vi "TCP Loop.vi"(8 "error in":errorcluster, 10 "Queues":T1, 11 "Notifiers":T2) -> (0 "error out":errorcluster)   [LabVIEW 2016, in "TCP.lvlib"]
uses:
  TCP.lvlib
  Support/Notifiers/Notifiers.ctl
  Support/Message Queue/All Message Queues.ctl
  Support/Message Queue/Message Cluster.ctl
  TypeDefs/TCP Data.ctl
  Support/Global names.vi
  Support/Message Queue/Enqueue Message (Single).vi
  <vilib>/Utility/error.llb/Error Cluster From Error Code.vi
  <vilib>/ErrorRing/Error Ring.xnode
  support/Message Queue/Message Queue.lvlib
  Model/Model.lvlib
  PLC/PLC.lvlib
  Support/Notifiers/Notifiers.lvlib
panel:
  out "Message":string
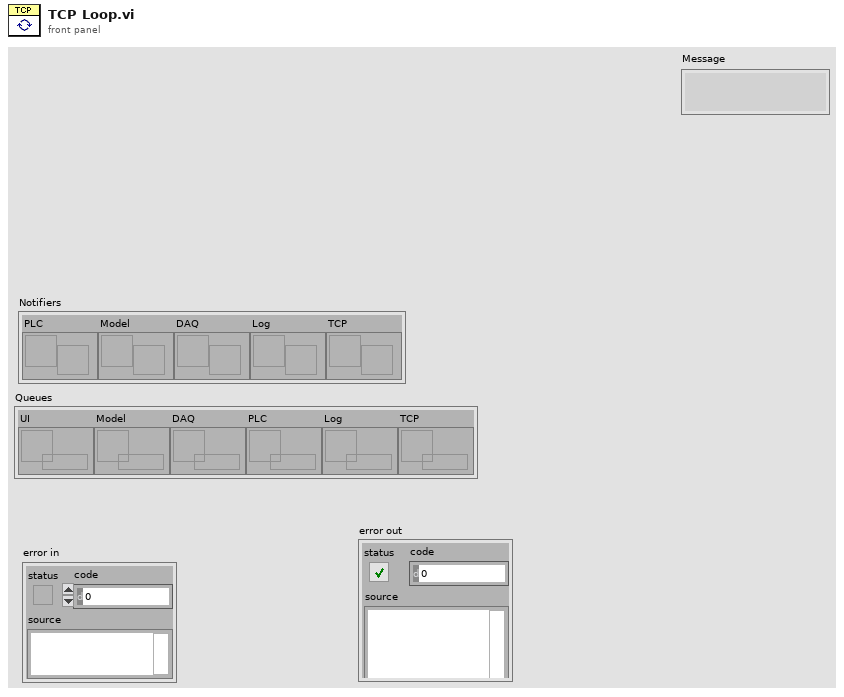
[diagram p1: front panel]
types:
  T1 = typedef "Message Queue.lvlib/All Message Queues.ctl" = cluster{"UI":refnum<queue>, "Model":refnum<queue>, "DAQ":refnum<queue>, "PLC":refnum<queue>, "Log":refnum<queue>, "TCP":refnum<queue>}
  T2 = typedef "Notifiers.lvlib/Notifiers.ctl" = cluster{"PLC":refnum<notifier>, "Model":refnum<notifier>, "DAQ":refnum<notifier>, "Log":refnum<notifier>, "TCP":refnum<notifier>}
  T3 = typedef "TCP.lvlib/TCP Data.ctl" = cluster{"Type":enum16{"Server", "Client"}, "IP":string, "Port":u16, "connection ID":refnum<k5>, "error":errorcluster, "Connected?":bool, "Data":string}
  T4 = enum16{"Standard", "Buffered", "CRLF", "Immediate"}
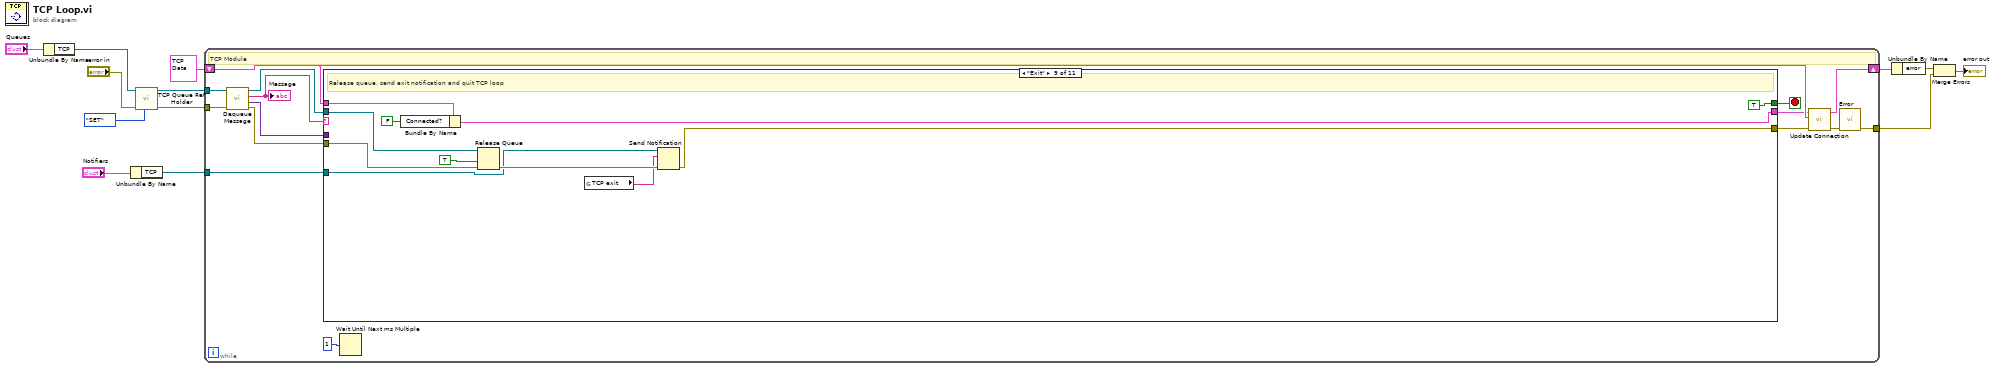
[diagram p0: block diagram]
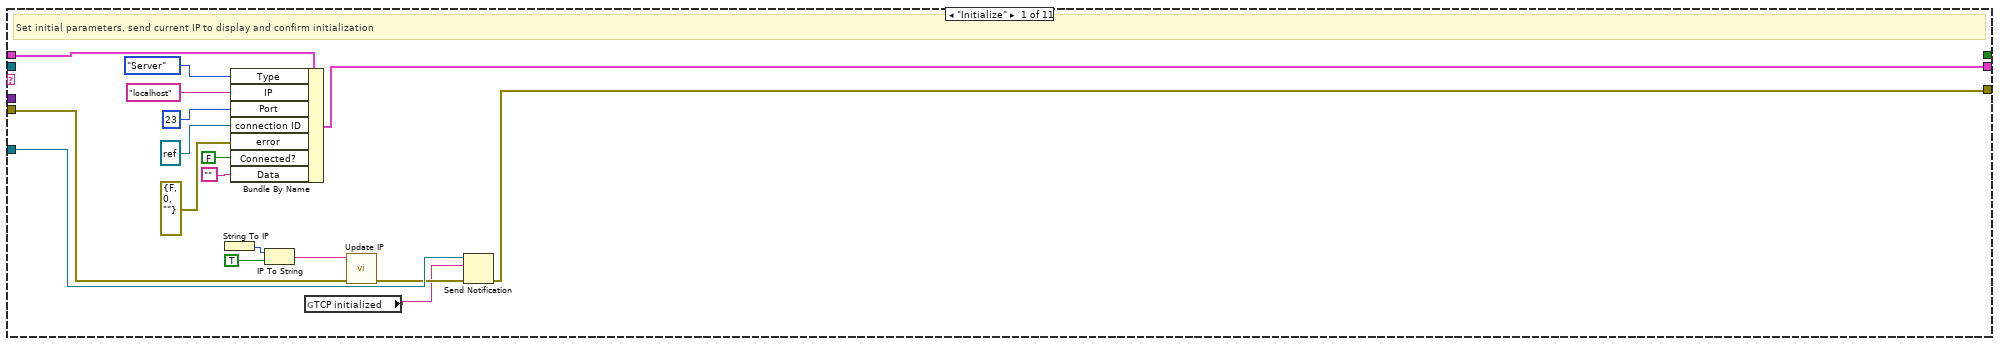
[diagram p2: hidden frame]
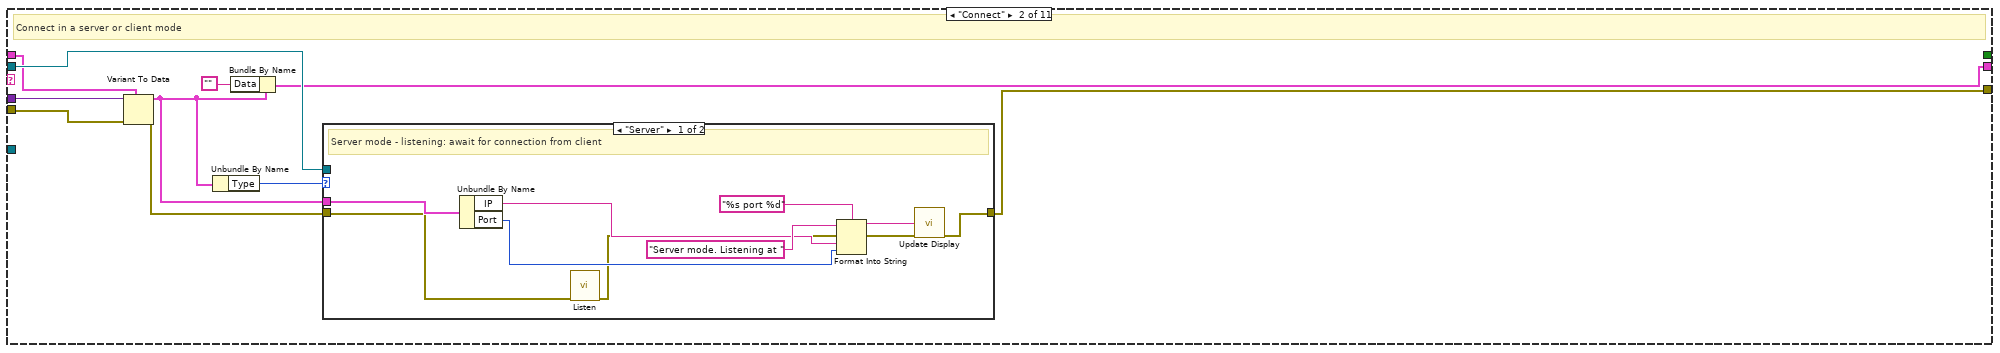
[diagram p3: hidden frame]
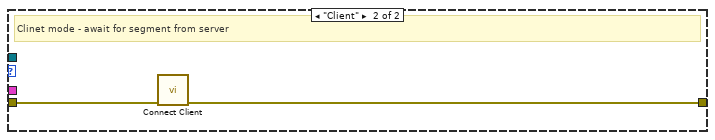
[diagram p4: hidden frame]
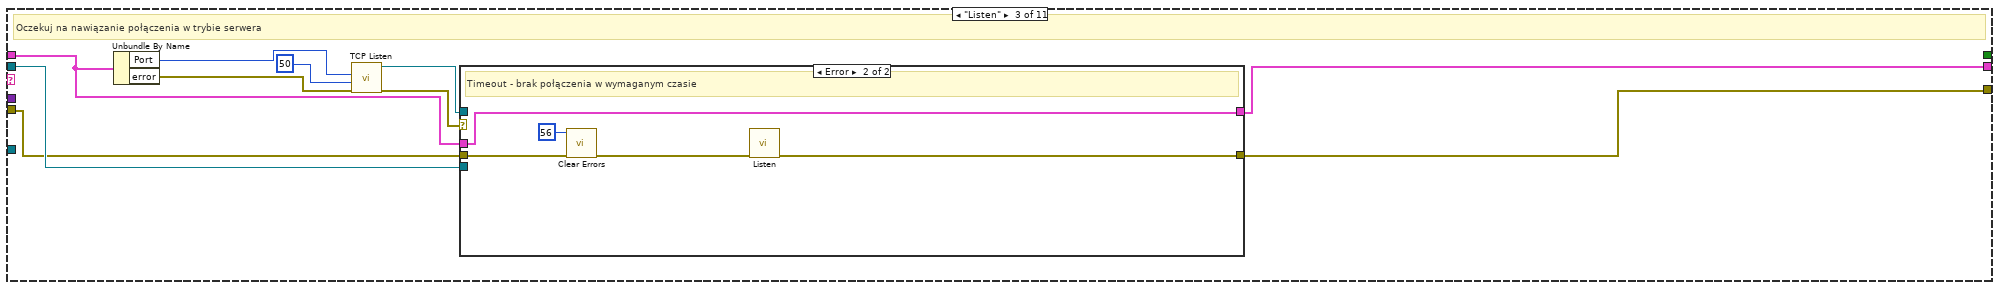
[diagram p5: hidden frame]
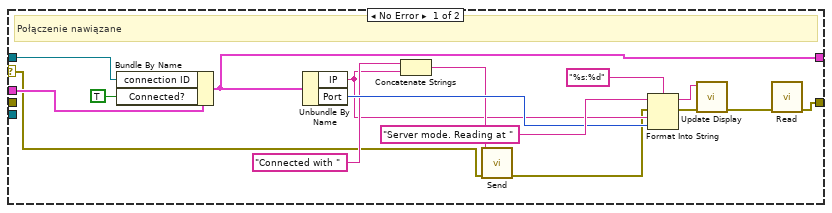
[diagram p6: hidden frame]
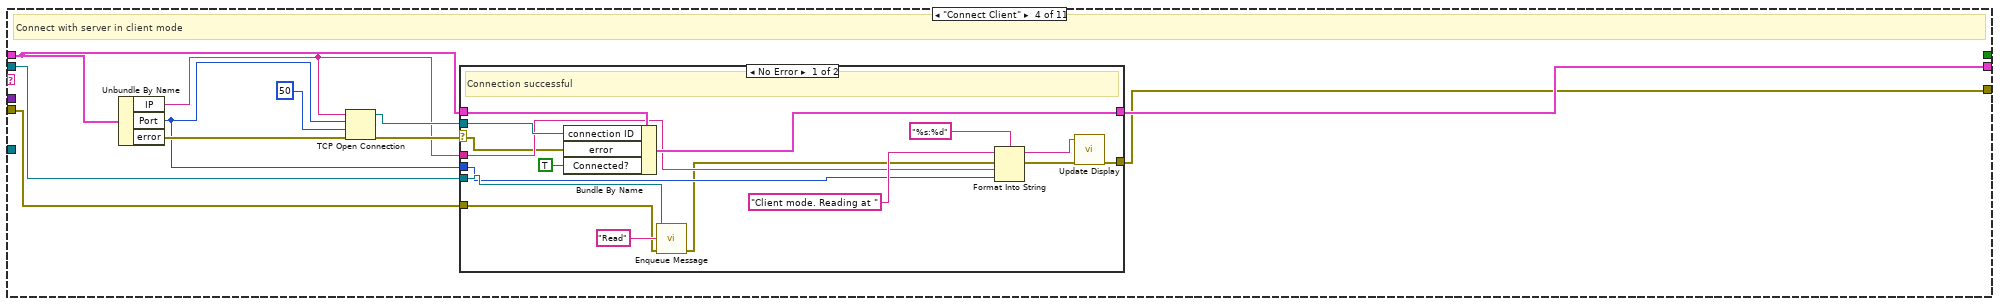
[diagram p7: hidden frame]
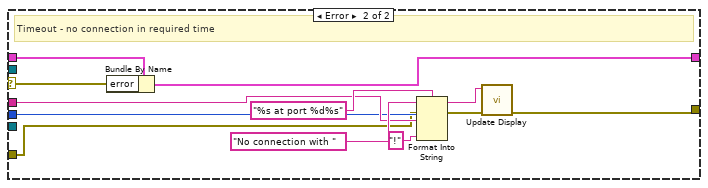
[diagram p8: hidden frame]
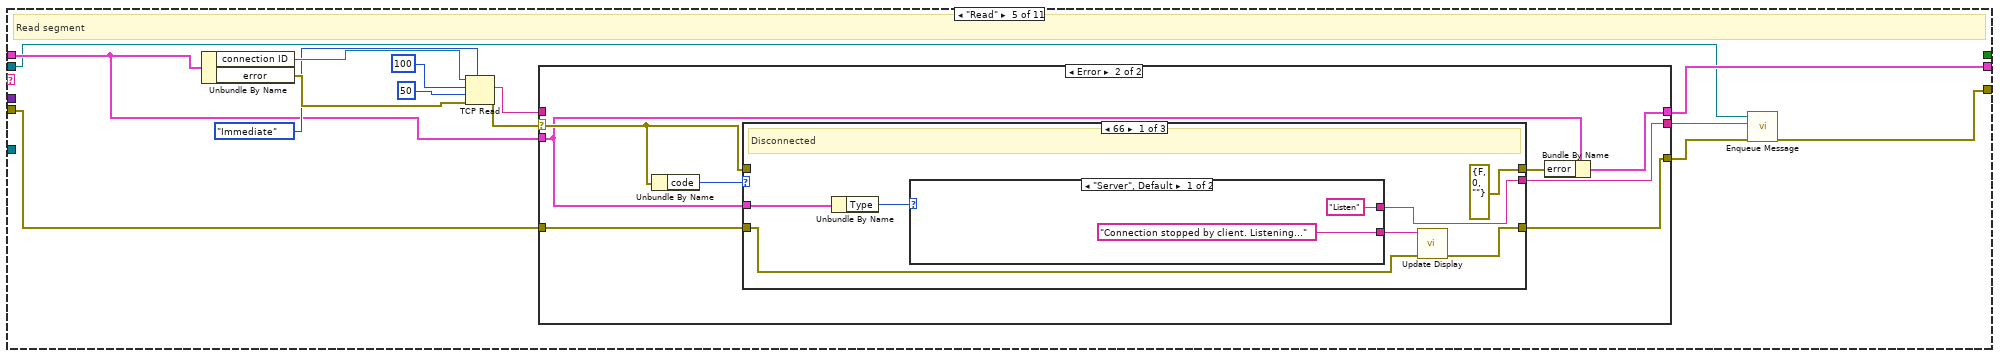
[diagram p9: hidden frame]
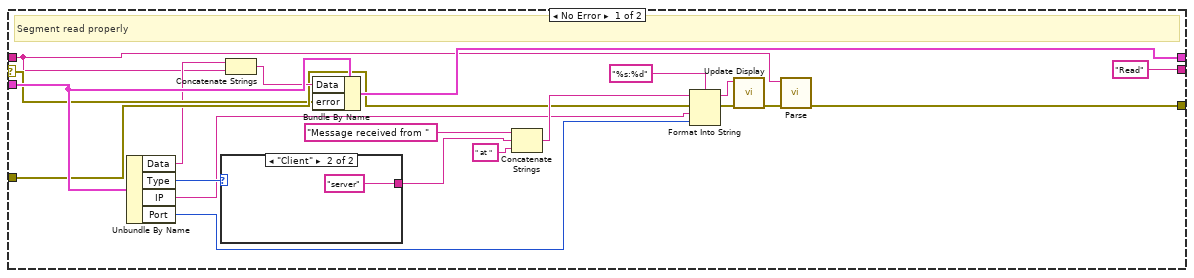
[diagram p10: hidden frame]
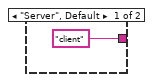
[diagram p11: hidden frame]
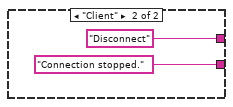
[diagram p12: hidden frame]
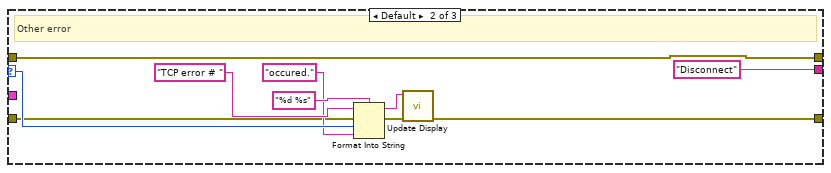
[diagram p13: hidden frame]
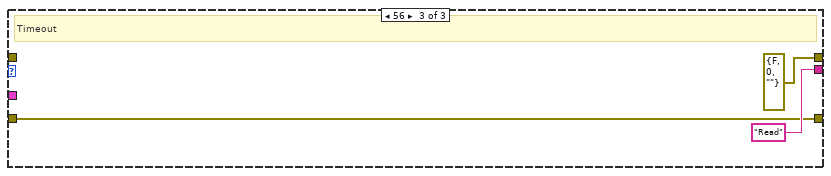
[diagram p14: hidden frame]
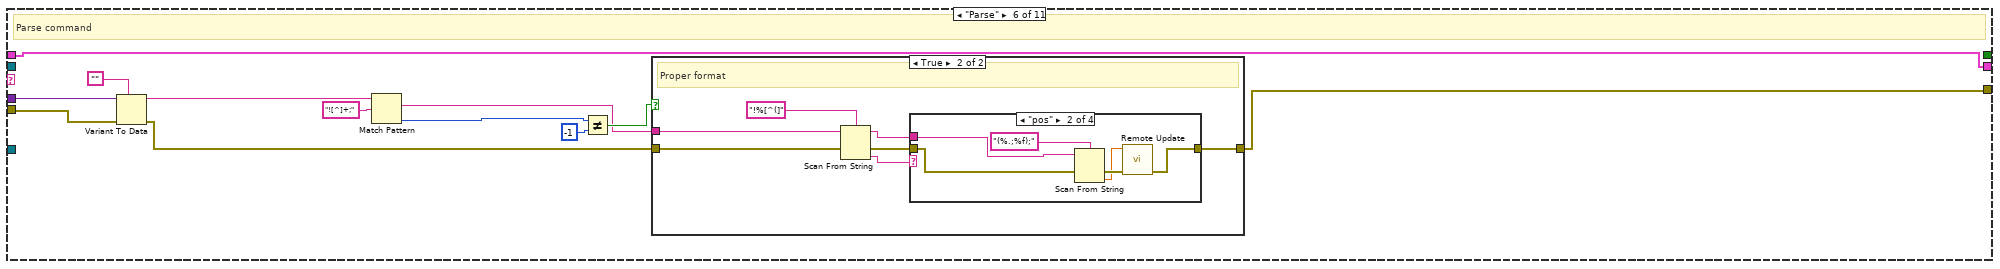
[diagram p15: hidden frame]
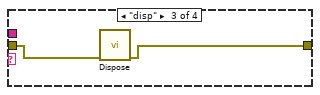
[diagram p18: hidden frame]
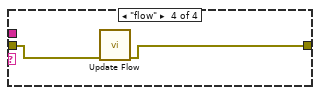
[diagram p19: hidden frame]
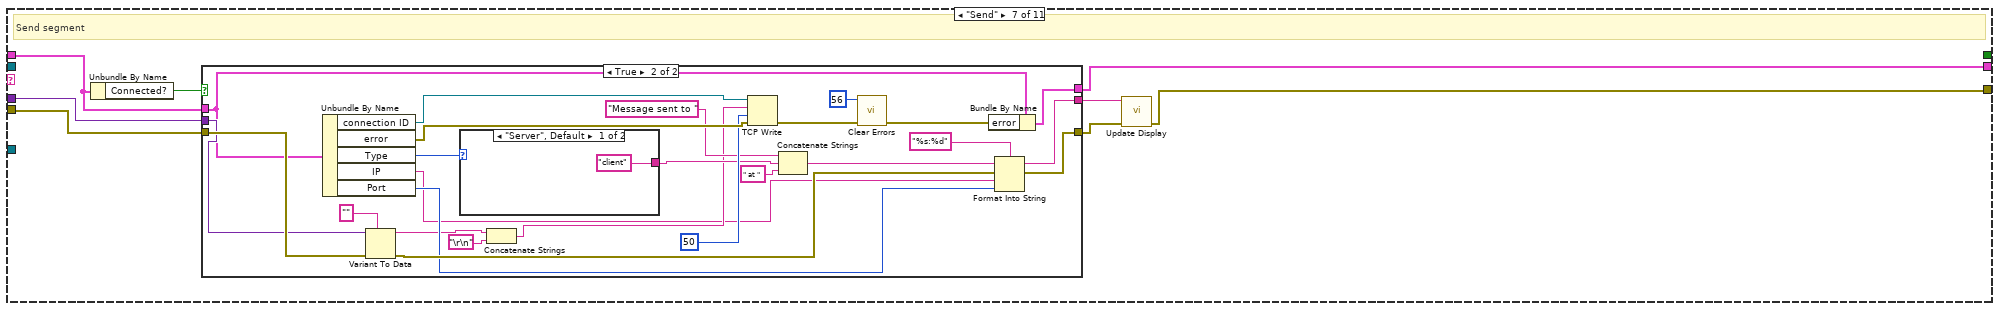
[diagram p20: hidden frame]
diagram:
  n1 = Unbundle By Name("Queues") -> ("TCP"=w2:refnum<queue>)
  n2 = Unbundle By Name("Notifiers") -> ("TCP"=w3:refnum<notifier>)
  n3 = call "TCP Queue Ref Holder.vi"("Action"=enum16{"GET", "SET"}."SET", "error in"="error in", "Message Queue In"=w2) -> ("error out"=w10:errorcluster, "Input Message Queue"=w12:refnum<queue>)  [unwired: 7 in]
  n4 = while {
    tunnel: w12 -> [w28]
    tunnel: w10 -> [w27]
    tunnel: [w17] -> w7
    tunnel: w3 -> [w22]
    shift-right: [w14] -> w9
    shift-left: T3 {"Type"=enum."Server", "IP"="", "Port"=0, "connection ID"=refnum, "error"={"status"=FALSE, "code"=0, "source"=""}, "Connected?"=FALSE, "Data"=""} ("TCP Data") -> [w16]
    stop <- w23 stop-if-true
    # "TCP Module"
    n5 = call "Dequeue Message.vi"("error in (no error)"=w27, "Message Queue"=w28) -> ("error out"=w25:errorcluster, "Message Data"=w21:variant, "Message"=w26:string, "dup Message Queue"=w24:refnum<queue>)  [unwired: 6 in]
    "Message" <- w26
    n6 = case shown="\"Exit\"" w26 {
      selector: w26 -> [_ _ _ _ _ _ _ _ _ w301 _]
      tunnel: w25 -> [w32 w54 w68 w102 w142 w215 w244 w286 w298 _ w312]
      tunnel: [w34 w53 w72 w101 w139 w206 w238 w276 w294 w300 w313] -> w20
      tunnel: w24 -> [_ w55 w73 w103 w138 _ _ w285 w297 _ _]
      tunnel: [_ _ _ _ _ _ _ _ TRUE _ _] -> w23
      tunnel: w22 -> [w33 _ _ _ _ _ _ _ w292 _ _]
      tunnel: w16 -> [w45 w51 w70 w105 w143 w212 w241 w284 w290 w299 w311]
      tunnel: [w44 w50 w69 w104 w141 w212 w242 w287 w289 w299 w311] -> w15
      tunnel: w21 -> [_ w52 _ _ _ w217 w243 _ _ _ _]
      frame "Initialize" {
        # "Set initial parameters, send current IP to display and confirm initialization"
        n7 = String To IP() -> (0:w35:u32)  [unwired: 1 in]
        n8 = Bundle By Name(cluster=w45, "Type"=enum16{"Server", "Client"}."Server", "IP"="localhost", "Port"=u16 23, "connection ID"=refnum<k5> refnum, "error"=errorcluster {"status"=FALSE, "code"=0, "source"=""}, "Connected?"=FALSE, "Data"="") -> (w44:T3)
        n9 = IP To String(1:TRUE ("dot notation? (F)"), 2:w35) -> (0:w30:string)
        n10 = global read "Global names.vi" "TCP initialized"() -> (w29:string)
        n11 = call "Update IP.vi"("error in"=w32, "Message string"=w30) -> ("error out"=w31:errorcluster)  [unwired: 9 in]
        n12 = Send Notification(notification=w29, notifier=w33, error in (no error)=w31) -> (error out=w34:errorcluster)  [unwired: 1 out]
      }
      frame "Connect" {
        # "Connect in a server or client mode"
        n13 = Variant To Data(error in=w54, type=w51, Variant=w52) -> (data=w46:T3, error out=w49:errorcluster)
        n14 = Unbundle By Name(w46) -> ("Type"=w48:enum16{"Server", "Client"})
        n15 = Bundle By Name(cluster=w46, "Data"="") -> (w50:T3)
        n16 = case shown="\"Server\"" w48 {
          tunnel: w55 -> [_ _]
          tunnel: w49 -> [w57 w67]
          tunnel: [w59 w66] -> w53
          tunnel: w46 -> [w61 _]
          frame "Server" {
            # "Server mode - listening: await for connection from client"
            n17 = Unbundle By Name(w61) -> ("IP"=w62:string, "Port"=w63:u16)
            n18 = call "Listen.vi"("error in"=w57) -> ("error out"=w56:errorcluster)  [unwired: 10 in]
            n19 = Format Into String(format string="%s port %d", initial string="Server mode. Listening at " ("Message"), error in=w56, w62, w63) -> (resulting string=w58:string, error out=w60:errorcluster)
            n20 = call "Update Display.vi"("error in"=w60, "Message string"=w58) -> ("error out"=w59:errorcluster)  [unwired: 9 in]
          }
          frame "Client" {
            # "Clinet mode - await for segment from server"
            n21 = call "Connect Client.vi"("error in"=w67) -> ("error out"=w66:errorcluster)  [unwired: 10 in]
          }
        }
      }
      frame "Listen" {
        # "Oczekuj na nawiązanie połączenia w trybie serwera"
        n22 = Unbundle By Name(w70) -> ("Port"=w77:u16, "error"=w75:errorcluster)
        n23 = call <vilib>:"TCP Listen.vi"("error in (no error)"=w75, "timeout ms (wait forever: -1)"=50, "port"=w77) -> ("error out"=w74:errorcluster, "connection ID"=w71:refnum<k5>)  [unwired: 4 in, 3 out]
        n24 = case shown="Error" w74 {
          selector: w74 -> [w83 _]
          tunnel: w73 -> [_ _]
          tunnel: [w78 w95] -> w72
          tunnel: w71 -> [w92 _]
          tunnel: w70 -> [w93 w96]
          tunnel: [w84 w96] -> w69
          tunnel: w68 -> [_ w98]
          frame No Error {
            # "Połączenie nawiązane"
            n25 = Bundle By Name(cluster=w93, "connection ID"=w92, "Connected?"=TRUE) -> (w84:T3)
            n26 = Unbundle By Name(w84) -> ("IP"=w85:string, "Port"=w88:u16)
            n27 = Concatenate Strings("Connected with " ("string"), w85) -> (w87:string)
            n28 = call "Send.vi"("error in"=w83, "Data"=w87) -> ("error out"=w82:errorcluster)  [unwired: 9 in]
            n29 = Format Into String(format string="%s:%d", initial string="Server mode. Reading at " ("Message"), error in=w82, w85, w88) -> (resulting string=w80:string, error out=w81:errorcluster)
            n30 = call "Update Display.vi"("error in"=w81, "Message string"=w80) -> ("error out"=w79:errorcluster)  [unwired: 9 in]
            n31 = call "Read.vi"("error in"=w79) -> ("error out"=w78:errorcluster)  [unwired: 10 in]
          }
          frame Error {
            # "Timeout - brak połączenia w wymaganym czasie"
            n32 = call <vilib>:"Clear Errors.vi"("error in (no error)"=w98, "specific error code to clear (0: all)"=56) -> ("error out"=w94:errorcluster)  [unwired: 4 in, 1 out]
            n33 = call "Listen.vi"("error in"=w94) -> ("error out"=w95:errorcluster)  [unwired: 10 in]
          }
        }
      }
      frame "Connect Client" {
        # "Connect with server in client mode"
        n34 = Unbundle By Name(w105) -> ("IP"=w100:string, "Port"=w99:u16, "error"=w108:errorcluster)
        n35 = TCP Open Connection(address=w100, remote port or service name=w99, timeout ms (60000)=50, error in (no error)=w108) -> (connection ID=w106:refnum<k5>, error out=w107:errorcluster)  [unwired: 1 in]
        n36 = case shown="No Error" w107 {
          selector: w107 -> [w113 w131]
          tunnel: [w122 w136] -> w104
          tunnel: w106 -> [w124 _]
          tunnel: w105 -> [w125 w137]
          tunnel: w102 -> [w114 w130]
          tunnel: w103 -> [w121 _]
          tunnel: [w111 w127] -> w101
          tunnel: w100 -> [w117 w133]
          tunnel: w99 -> [w116 w132]
          frame No Error {
            # "Connection successful"
            n37 = Bundle By Name(cluster=w125, "connection ID"=w124, "error"=w113, "Connected?"=TRUE) -> (w122:T3)
            n38 = call-poly "Enqueue Message.vi"("error in (no error)"=w114, "Message"="Read", "Message Queue"=w121) -> ("error out"=w115:errorcluster)  [unwired: 7 in, 1 out]
            n39 = Format Into String(format string="%s:%d", initial string="Client mode. Reading at " ("Message"), error in=w115, w117, w116) -> (resulting string=w110:string, error out=w112:errorcluster)
            n40 = call "Update Display.vi"("error in"=w112, "Message string"=w110) -> ("error out"=w111:errorcluster)  [unwired: 9 in]
          }
          frame Error {
            # "Timeout - no connection in required time"
            n41 = Bundle By Name(cluster=w137, "error"=w131) -> (w136:T3)
            n42 = Format Into String(format string="%s at port %d%s", initial string="No connection with " ("Message"), error in=w130, w133, w132, "!" ("input 3")) -> (resulting string=w126:string, error out=w128:errorcluster)
            n43 = call "Update Display.vi"("error in"=w128, "Message string"=w126) -> ("error out"=w127:errorcluster)  [unwired: 9 in]
          }
        }
      }
      frame "Read" {
        # "Read segment"
        n44 = Unbundle By Name(w143) -> ("connection ID"=w151:refnum<k5>, "error"=w148:errorcluster)
        n45 = TCP Read(connection ID=w151, bytes to read=100, error in (no error)=w148, 7:T4."Immediate" ("mode (standard)"), 9:50 ("timeout ms (25000)")) -> (data out=w144:string, error out=w146:errorcluster)  [unwired: 1 out]
        n46 = case shown="Error" w146 {
          selector: w146 -> [w158 w179]
          tunnel: [w170 w178] -> w141
          tunnel: ["Read" ("Message") w180] -> w145
          tunnel: w144 -> [w153 _]
          tunnel: w143 -> [w169 w176]
          tunnel: w142 -> [w161 w175]
          tunnel: [w152 w174] -> w140
          frame No Error {
            # "Segment read properly"
            n47 = Unbundle By Name(w169) -> ("Data"=w157:string, "Type"=w163:enum16{"Server", "Client"}, "IP"=w159:string, "Port"=w162:u16)
            n48 = case shown="\"Client\"" w163 {
              tunnel: ["client" ("Message") "server" ("f")] -> w160
              frame "Server", Default {
              }
              frame "Client" {
              }
            }
            n49 = Concatenate Strings(w157, w153) -> (w168:string)
            n50 = Bundle By Name(cluster=w169, "Data"=w168, "error"=w158) -> (w170:T3)
            n51 = Concatenate Strings("Message received from " ("Message"), w160, " at " ("string")) -> (w166:string)
            n52 = Format Into String(format string="%s:%d", initial string=w166, error in=w161, w159, w162) -> (resulting string=w155:string, error out=w156:errorcluster)
            n53 = call "Update Display.vi"("error in"=w156, "Message string"=w155) -> ("error out"=w154:errorcluster)  [unwired: 9 in]
            n54 = call "Parse.vi"("error in"=w154, "String"=w153) -> ("error out"=w152:errorcluster)  [unwired: 9 in]
          }
          frame Error {
            n55 = Unbundle By Name(w179) -> ("code"=w181:i32)
            n56 = case shown="66" w181 {
              selector: w181 -> [_ w198 _]
              tunnel: [w185 "Disconnect" ("Message") "Read" ("Message")] -> w180
              tunnel: w179 -> [_ w202 _]
              tunnel: [errorcluster {"status"=FALSE, "code"=0, "source"=""} ("error") w202 errorcluster {"status"=FALSE, "code"=0, "source"=""} ("error")] -> w177
              tunnel: w176 -> [w187 _ _]
              tunnel: w175 -> [w184 w196 w203]
              tunnel: [w183 w194 w203] -> w174
              frame 66 {
                # "Disconnected"
                n57 = Unbundle By Name(w187) -> ("Type"=w186:enum16{"Server", "Client"})
                n58 = case shown="\"Server\", Default" w186 {
                  tunnel: ["Listen" ("Message") "Disconnect" ("Message")] -> w185
                  tunnel: ["Connection stopped by client. Listening..." ("Message") "Connection stopped." ("Message")] -> w182
                  frame "Server", Default {
                  }
                  frame "Client" {
                  }
                }
                n59 = call "Update Display.vi"("error in"=w184, "Message string"=w182) -> ("error out"=w183:errorcluster)  [unwired: 9 in]
              }
              frame Default {
                # "Other error"
                n60 = Format Into String(format string="%d %s", initial string="TCP error # " ("Message"), error in=w196, w198, "occured." ("input 2")) -> (resulting string=w193:string, error out=w195:errorcluster)
                n61 = call "Update Display.vi"("error in"=w195, "Message string"=w193) -> ("error out"=w194:errorcluster)  [unwired: 9 in]
              }
              frame 56 {
                # "Timeout"
              }
            }
            n62 = Bundle By Name(cluster=w176, "error"=w177) -> (w178:T3)
          }
        }
        n63 = call-poly "Enqueue Message.vi"("error in (no error)"=w140, "Message"=w145, "Message Queue"=w138) -> ("error out"=w139:errorcluster)  [unwired: 7 in, 1 out]
      }
      frame "Parse" {
        # "Parse command"
        n64 = Variant To Data(error in=w215, type="", Variant=w217) -> (data=w214:string, error out=w207:errorcluster)
        n65 = Match Pattern(string=w214, regular expression="![^]+;") -> (match substring=w208:string, offset past match=w211:i32)  [unwired: 1 in, 2 out]
        n66 = Not Equal?(x=w211, y=-1) -> (x != y?=w209:bool)
        n67 = case shown="True" w209 {
          tunnel: w208 -> [_ w225]
          tunnel: w207 -> [w218 w224]
          tunnel: [w218 w220] -> w206
          frame False {
            # "Incorrect format"
          }
          frame True {
            # "Proper format"
            n68 = Scan From String(format string="!%[^(]", input string=w225, error in=w224) -> (remaining string=w219:string, error out=w221:errorcluster, output 1=w222:string)  [unwired: 2 in, 1 out]
            n69 = case shown="\"pos\"" w222 {
              tunnel: w221 -> [w226 w230 w234 w236]
              tunnel: [w226 w228 w233 w235] -> w220
              tunnel: w219 -> [_ w231 _ _]
              frame Default {
              }
              frame "pos" {
                n70 = Scan From String(format string="(%.;%f);", input string=w231, error in=w230) -> (error out=w229:errorcluster, output 1=w227:dbl)  [unwired: 2 in, 2 out]
                n71 = call "Remote Update.vi"("error in"=w229, "Value"=w227) -> ("error out"=w228:errorcluster)  [unwired: 9 in]
              }
              frame "disp" {
                n72 = call "Dispose.vi"("error in (no error)"=w234) -> ("error out"=w233:errorcluster)  [unwired: 10 in]
              }
              frame "flow" {
                n73 = call "Update Flow.vi"("error in (no error)"=w236) -> ("error out"=w235:errorcluster)  [unwired: 10 in]
              }
            }
          }
        }
      }
      frame "Send" {
        # "Send segment"
        n74 = Unbundle By Name(w241) -> ("Connected?"=w240:bool)
        n75 = case shown="True" w240 {
          tunnel: w244 -> [w246 w270]
          tunnel: w243 -> [_ w269]
          tunnel: w241 -> [w245 w267]
          tunnel: [w245 w248] -> w242
          tunnel: ["No connection - data not sent!" w262] -> w237
          tunnel: [w246 w261] -> w239
          frame False {
          }
          frame True {
            n76 = Unbundle By Name(w267) -> ("connection ID"=w272:refnum<k5>, "error"=w271:errorcluster, "Type"=w257:enum16{"Server", "Client"}, "IP"=w251:string, "Port"=w254:u16)
            n77 = Variant To Data(error in=w270, type="", Variant=w269) -> (data=w250:string, error out=w260:errorcluster)
            n78 = case shown="\"Server\", Default" w257 {
              tunnel: ["client" ("Message") "server" ("f")] -> w256
              frame "Server", Default {
              }
              frame "Client" {
              }
            }
            n79 = Concatenate Strings(w250, "\r\n") -> (w252:string)
            n80 = TCP Write(connection ID=w272, data in=w252, error in (no error)=w271, 9:50 ("timeout ms (25000)")) -> (error out=w266:errorcluster)  [unwired: 2 out]
            n81 = Concatenate Strings("Message sent to " ("Message"), w256, " at " ("string")) -> (w258:string)
            n82 = call <vilib>:"Clear Errors.vi"("error in (no error)"=w266, "specific error code to clear (0: all)"=56) -> ("error out"=w265:errorcluster)  [unwired: 4 in, 1 out]
            n83 = Bundle By Name(cluster=w267, "error"=w265) -> (w248:T3)
            n84 = Format Into String(format string="%s:%d", initial string=w258, error in=w260, w251, w254) -> (resulting string=w262:string, error out=w261:errorcluster)
          }
        }
        n85 = call "Update Display.vi"("error in"=w239, "Message string"=w237) -> ("error out"=w238:errorcluster)  [unwired: 9 in]
      }
      frame "Disconnect" {
        # "Disconnect"
        n86 = Unbundle By Name(w284) -> ("connection ID"=w283:refnum<k5>, "error"=w280:errorcluster)
        n87 = Flush Queue(queue=w285, error in (no error)=w286) -> (error out=w277:errorcluster)  [unwired: 2 out]
        n88 = TCP Close Connection(connection ID=w283, error in (no error)=w280) -> (error out=w279:errorcluster)  [unwired: 1 in, 1 out]
        n89 = call <vilib>:"Clear Errors.vi"("error in (no error)"=w279) -> ("error out"=w278:errorcluster)  [unwired: 5 in, 1 out]
        n90 = call "Update Display.vi"("error in"=w277, "Message string"="Connection closed." ("Message")) -> ("error out"=w276:errorcluster)  [unwired: 9 in]
        n91 = Bundle By Name(cluster=w284, "connection ID"=refnum<k5> refnum, "error"=w278, "Connected?"=FALSE) -> (w287:T3)
      }
      frame "Exit" {
        # "Release queue, send exit notification and quit TCP loop"
        n92 = Bundle By Name(cluster=w290, "Connected?"=FALSE) -> (w289:T3)
        n93 = Release Queue(queue=w297, force destroy? (F)=TRUE, error in (no error)=w298) -> (error out=w295:errorcluster)  [unwired: 2 out]
        n94 = global read "Global names.vi" "TCP exit"() -> (w288:string)
        n95 = Send Notification(notification=w288, notifier=w292, error in (no error)=w295) -> (error out=w294:errorcluster)  [unwired: 1 out]
      }
      frame Default {
        # "Incorrect message"
        n96 = xnode "Error Ring"("parameter 0"=w301) -> ("error out"=w300:errorcluster)
      }
      frame "Say goodbye" {
        # "Send goodbye info"
        n97 = Unbundle By Name(w311) -> ("Connected?"=w309:bool, "IP"=w310:string)
        n98 = case shown="True" w309 {
          tunnel: [w314 w319] -> w313
          tunnel: w312 -> [w314 w318]
          tunnel: w310 -> [_ w316]
          frame False {
          }
          frame True {
            n99 = Concatenate Strings("Disconnected with " ("string"), w316) -> (w315:string)
            n100 = call "Send.vi"("error in"=w318, "Data"=w315) -> ("error out"=w319:errorcluster)  [unwired: 9 in]
          }
        }
      }
    }
    n101 = Wait Until Next ms Multiple(millisecond multiple=u32 1) -> ()  [unwired: 1 out]
    n102 = call "Update Connection.vi"("error in (no error)"=w20, "TCP Data before update"=w16, "TCP Data after update"=w15) -> ("error out"=w18:errorcluster, "TCP Data after update out"=w14:T3)  [unwired: 7 in]
    n103 = call "Error.vi"("error in"=w18) -> ("error out"=w17:errorcluster)  [unwired: 10 in]
  }
  n104 = Unbundle By Name(w9) -> ("error"=w8:errorcluster)
  n105 = Merge Errors(w8, w7) -> (→"error out":errorcluster)
